vi "今日-日期时间字符串.vi"() -> (0 "日期时间":string, 2 "hh:mm:ss":string, 3 "YYYY-MM-DD":string)   [LabVIEW 2013]
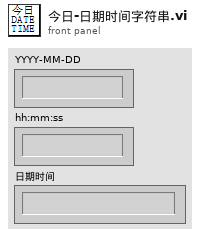
[diagram p1: front panel]
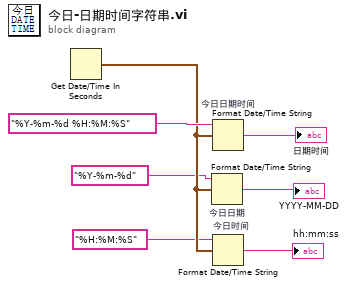
[diagram p0: block diagram]
diagram:
  n1 = Get Date/Time In Seconds() -> (seconds since 1Jan1904=w6:timestamp)
  n2 = Format Date/Time String "今日日期"(time format string (%c)="%Y-%m-%d" ("时间格式字符串(%c)"), seconds (now)=w6) -> (date/time string=→"YYYY-MM-DD":string)  [unwired: 1 in]
  n3 = Format Date/Time String "今日日期时间"(time format string (%c)="%Y-%m-%d %H:%M:%S" ("时间格式字符串(%c)"), seconds (now)=w6) -> (date/time string=→"日期时间":string)  [unwired: 1 in]
  n4 = Format Date/Time String "今日时间"(time format string (%c)="%H:%M:%S" ("时间格式字符串(%c)"), seconds (now)=w6) -> (date/time string=→"hh:mm:ss":string)  [unwired: 1 in]
